vi "Prepare data and write to file.vi"(0 "Photon time (ms)":dbl, 1 "String":string, 2 "Confidence":i32, 3 "Photon #":i32, 4 "Pump WP":dbl, 5 "Observer choice":string, 6 "LED Voltage":dbl, 7 "Response \ntime (ms)":dbl, 8 "Path in":path, 9 "Boolean":bool, 10 "?":i32, 11 "Counts in":u32, 12 "Subject #":string, 13 "Counts 1":u32) -> ()   [LabVIEW 2013]
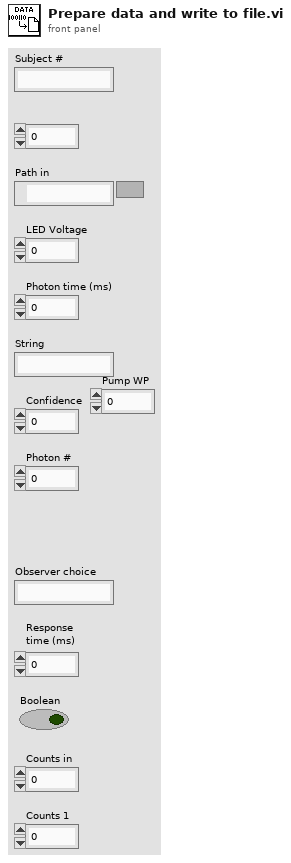
[diagram p1: front panel]
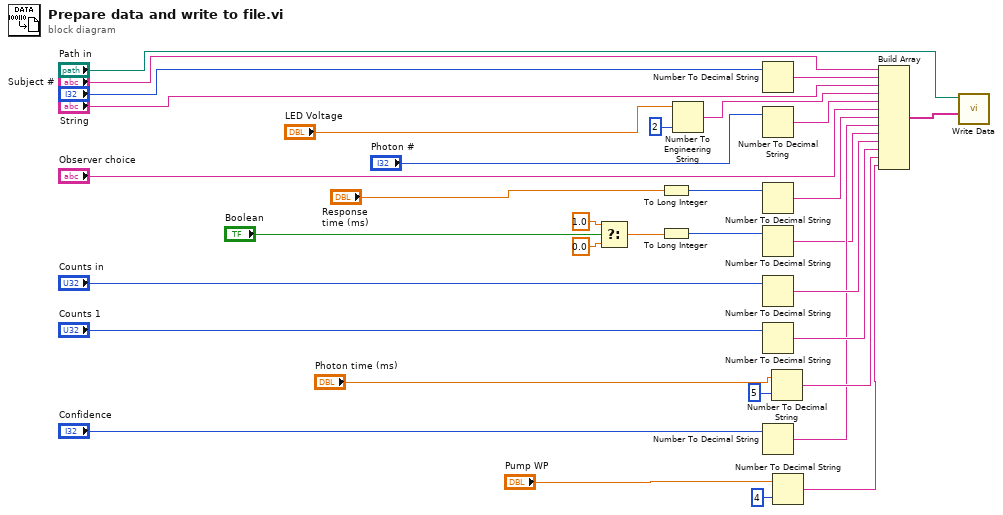
[diagram p0: block diagram]
diagram:
  n1 = Select(t=1.0, s="Boolean", f=0.0) -> (s? t:f=w8:dbl)
  n2 = To Long Integer(number="Response \ntime (ms)") -> (32bit integer=w13:i32)
  n3 = To Long Integer(number=w8) -> (32bit integer=w9:i32)
  n4 = Number To Engineering String(2:i16 2 ("width (-)"), 4:"LED Voltage") -> (0:w17:string)  [unwired: 2 in]
  n5 = Number To Decimal String(number="?") -> (decimal integer string=w26:string)  [unwired: 1 in]
  n6 = Number To Decimal String(number="Photon #") -> (decimal integer string=w28:string)  [unwired: 1 in]
  n7 = Number To Decimal String(number=w13) -> (decimal integer string=w14:string)  [unwired: 1 in]
  n8 = Number To Decimal String(number=w9) -> (decimal integer string=w10:string)  [unwired: 1 in]
  n9 = Number To Decimal String(number="Counts in") -> (decimal integer string=w22:string)  [unwired: 1 in]
  n10 = Number To Decimal String(number="Counts 1") -> (decimal integer string=w24:string)  [unwired: 1 in]
  n11 = Number To Decimal String(number="Confidence") -> (decimal integer string=w11:string)  [unwired: 1 in]
  n12 = Number To Decimal String(number="Photon time (ms)", width (-)=i16 5) -> (decimal integer string=w30:string)
  n13 = Number To Decimal String(number="Pump WP", width (-)=i16 4) -> (decimal integer string=w1:string)
  n14 = Build Array("Subject #", w26, "String", w17, w28, "Observer choice", w14, w11, w10, w22, w24, w30, w1) -> (w4:string[])
  n15 = call "Write Data.vi"("Trial Results"=w4, "base path"="Path in") -> ()  [unwired: 10 in]
